vi "Get Decimation.vi"(8 "error in":errorcluster, 11 "Ballard MIL-STD 1553 custom device in":T1 format="%.0x") -> (0 "error out":errorcluster, 2 "decimation":i32, 3 "Ballard MIL-STD 1553 custom device out":T1 format="%.0x")   [LabVIEW 2020, in "Ballard MIL-STD-1553 Scripting.lvlib"]
uses:
  Ballard MIL-STD-1553 Scripting.lvlib
  <vilib>/NI VeriStand/Custom Device API/Custom Device Item Ref.ctl
  <vilib>/NI VeriStand/Custom Device API/Custom Device API.lvlib
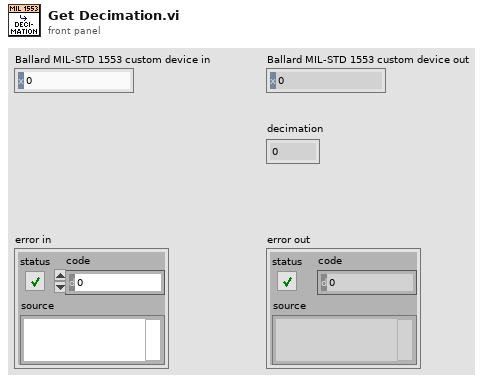
[diagram p1: front panel]
types:
  T1 = typedef "Custom Device API.lvlib/Custom Device Item Ref.ctl" = u64
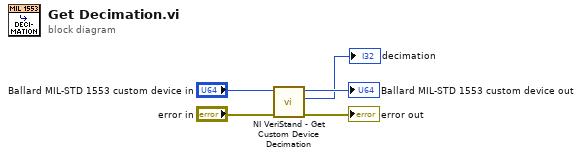
[diagram p0: block diagram]
diagram:
  n1 = call <vilib>:"NI VeriStand - Get Custom Device Decimation.vi"("error in (no error)"="error in", "Device Ref in"="Ballard MIL-STD 1553 custom device in") -> ("error out"=→"error out":errorcluster, "Decimation"=→"decimation":i32, "Device Ref out"=→"Ballard MIL-STD 1553 custom device out":T1)  [unwired: 7 in]
